vi "UI Cleanup.vi"(8 "error in (no error)":errorcluster) -> (0 "error out":errorcluster)   [LabVIEW 2017]
uses:
  Global Variables/gl_UI Ctrl Refs.vi
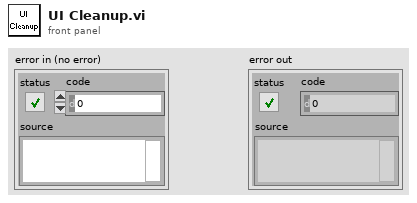
[diagram p1: front panel]
types:
  T1 = enum8{"Enabled", "Disabled", "Disabled and Grayed Out"}
  T2 = typedef "UI ctrl refs cluster.ctl" = cluster{"Top level VI path":path, "Top level VI ref":refnum<vi>, "User menu ref":refnum<k9>, "Sub Panel control":refnum<vi>, "Imaging Param Tab":refnum<vi>, "Occurrence-Start drivers":refnum<k4>, "Occurrence-Speed logging initialised":refnum<k4>, "Occurrence-XYZ stage initialised":refnum<k4>, "Exit button":refnum<vi>, "Status ind":refnum<vi>, "Set as origin":refnum<vi>, "Speed Logging":refnum<vi>, "Time Lapse":refnum<vi>, "Live Imaging":refnum<vi>, "AOL Z Stack":refnum<vi>, "Motor Z Stack":refnum<vi>, "Funct Acq button":refnum<vi>, "Hard Shutter":refnum<vi>, "Virtual Shutter":refnum<vi>, "Laser Power":refnum<vi>, "AOL Mode":refnum<vi>, "Frame Size":refnum<vi>, "Field of View":refnum<vi>, "Dwell Time":refnum<vi>, "Zoom":refnum<vi>, "AOL Z":refnum<vi>, "Objective":refnum<vi>, "Axis":refnum<vi>, "Paths & Names":refnum<vi>, "Experiment folder path (ind.)":refnum<vi>, "Last State (Ind.)":refnum<vi>, "Laser wavelength ind (nm)":refnum<vi>, "Averages":refnum<vi>, "Angle (degrees)":refnum<vi>, "X centre":refnum<vi>, "Y centre":refnum<vi>, "Plane Mode":refnum<vi>, "# Planes":refnum<vi>, "Z Start":refnum<vi>, "Z Stop":refnum<vi>, "Z Step":refnum<vi>, "PMT 1":refnum<vi>, "PMT 2":refnum<vi>, "Stage XYZ Position":refnum<vi>, "Pockels@Z Start":refnum<vi>, "Pockels@Z Stop":refnum<vi>, "Obtain Z Start":refnum<vi>, "Obtain Z Stop":refnum<vi>, "Live stim.trig.period":refnum<vi>, "Live stim.trig.enable":refnum<vi>, "Movement Correction":refnum<vi>, "Load Reference Image":refnum<vi>, "XY Stage Move":refnum<vi>, "MovCor Cluster":refnum<vi>, "RefDAQParam":refnum<vi>, "Funct. Acq. Pockels Modulation":refnum<vi>, "Background MovCor":refnum<vi>, "Ref Laser Power":refnum<vi>, "Enable Video Recording":refnum<vi>, "Video Record-Live Imaging":refnum<vi>, "Video Record-Funct acq":refnum<vi>, "Reference Source":refnum<vi>, "AOL Z-stack Chirps Ready (ind)":refnum<vi>, "Target time between mov.cor. ref triggers (ms)":refnum<vi>, "Funct. Acq. Ref frame save":refnum<vi>, "Tracking button":refnum<vi>, "Show ref plots window":refnum<vi>, "Center freq ind (nm)":refnum<vi>, "Pickup mode (ind)":refnum<vi>, "Logging queue (ind)":refnum<vi>, "Back aperture power (ind.)":refnum<vi>, "Power after objective (ind.)":refnum<vi>, "Switch user":refnum<vi>}
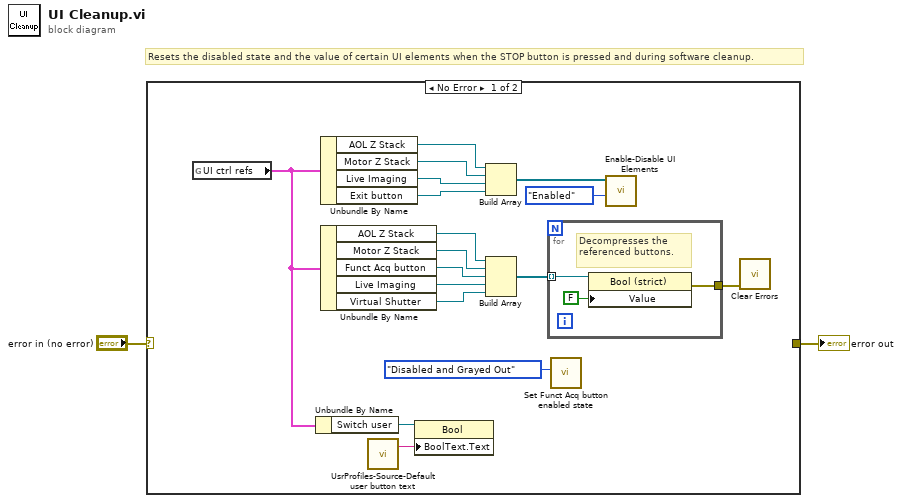
[diagram p0: block diagram]
diagram:
  # "Resets the disabled state and the value of certain UI elements when the STOP button is pressed and during software cleanup."
  n1 = case shown="No Error" "error in (no error)" {
    selector: "error in (no error)" -> [_ w23]
    tunnel: [_ w23] -> w1
    frame No Error {
      n2 = global read "gl_UI Ctrl Refs.vi" "UI ctrl refs"() -> (w5:T2)
      n3 = Unbundle By Name(w5) -> ("Switch user"=w4:refnum<vi>)
      n4 = Unbundle By Name(w5) -> ("AOL Z Stack"=w11:refnum<vi>, "Motor Z Stack"=w9:refnum<vi>, "Live Imaging"=w10:refnum<vi>, "Exit button"=w12:refnum<vi>)
      n5 = Unbundle By Name(w5) -> ("AOL Z Stack"=w15:refnum<vi>, "Motor Z Stack"=w18:refnum<vi>, "Funct Acq button"=w17:refnum<vi>, "Live Imaging"=w16:refnum<vi>, "Virtual Shutter"=w7:refnum<vi>)
      n6 = call "UsrProfiles-Source-Default user button text.vi"() -> ("Default user boolean text constant"=w3:string)  [unwired: 3 in]
      n7 = property class="Bool"(reference=w4, "BoolText.Text"=w3) -> ()  [unwired: 1 in, 2 out]
      n8 = Build Array(w11, w9, w10, w12) -> (w14:refnum<vi>[])
      n9 = Build Array(w15, w18, w17, w16, w7) -> (w19:refnum<vi>[])
      n10 = for {
        tunnel: w19 -> [w22] mode=indexing
        tunnel: [w20] -> w8
        # "Decompresses the referenced buttons."
        n11 = property class="Bool (strict)"(reference=w22, "Value"=FALSE) -> (error out=w20:errorcluster)  [unwired: 1 in, 1 out]
      }
      n12 = call "Set Funct Acq button enabled state.vi"("Disabled"=T1."Disabled and Grayed Out") -> ()  [unwired: 10 in, 1 out]
      n13 = call "Enable-Disable UI Elements.vi"("Enable/Disable"=T1."Enabled", "Ctrl ref's"=w14) -> ()  [unwired: 9 in, 1 out]
      n14 = call <vilib>:"Clear Errors.vi"("error in (no error)"=w8) -> ()  [unwired: 5 in, 2 out]
    }
    frame Error {
    }
  }
  "error out" <- w1
